vi "get user path.vi"(8 "error in":errorcluster) -> (0 "error out":errorcluster, 3 "Path":path)   [LabVIEW 2013]
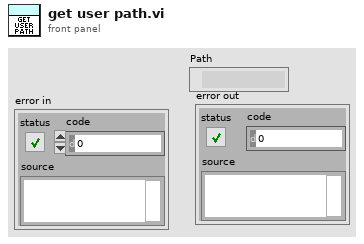
[diagram p1: front panel]
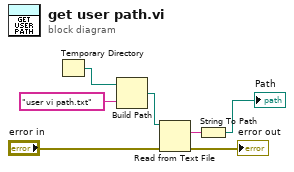
[diagram p0: block diagram]
diagram:
  n1 = Temporary Directory() -> (w1:path)
  n2 = Build Path(base path=w1, name or relative path="user vi path.txt") -> (appended path=w5:path)
  n3 = Read from Text File(file (use dialog)=w5, error in="error in") -> (text=w6:string, error out=→"error out":errorcluster)  [unwired: 2 in, 2 out]
  n4 = String To Path(string=w6) -> (path=→"Path":path)
